vi "Set Worker.vi"(7 "Worker VI Path":path, 9 "State In":T1) -> (1 "State":T1, 2 "Is Worker?":bool)   [LabVIEW 2020, in "FlexBlock.xnode"]
uses:
  FlexBlock.xnode
  FlexBlocks/Terminal Direction.ctl
  FlexBlocks/FlexBlocks.lvlib
  FlexBlocks/Value Mode.ctl
  FlexBlocks/Terminal State.ctl
  FlexBlocks/Type Descriptor.ctl
  FlexBlocks/Errors.ctl
  <vilib>/picture/picture.llb/imagedata.ctl
  State.ctl
  FlexBlocks/Special Terminal.ctl
  FlexBlocks/Calculated Sizes.ctl
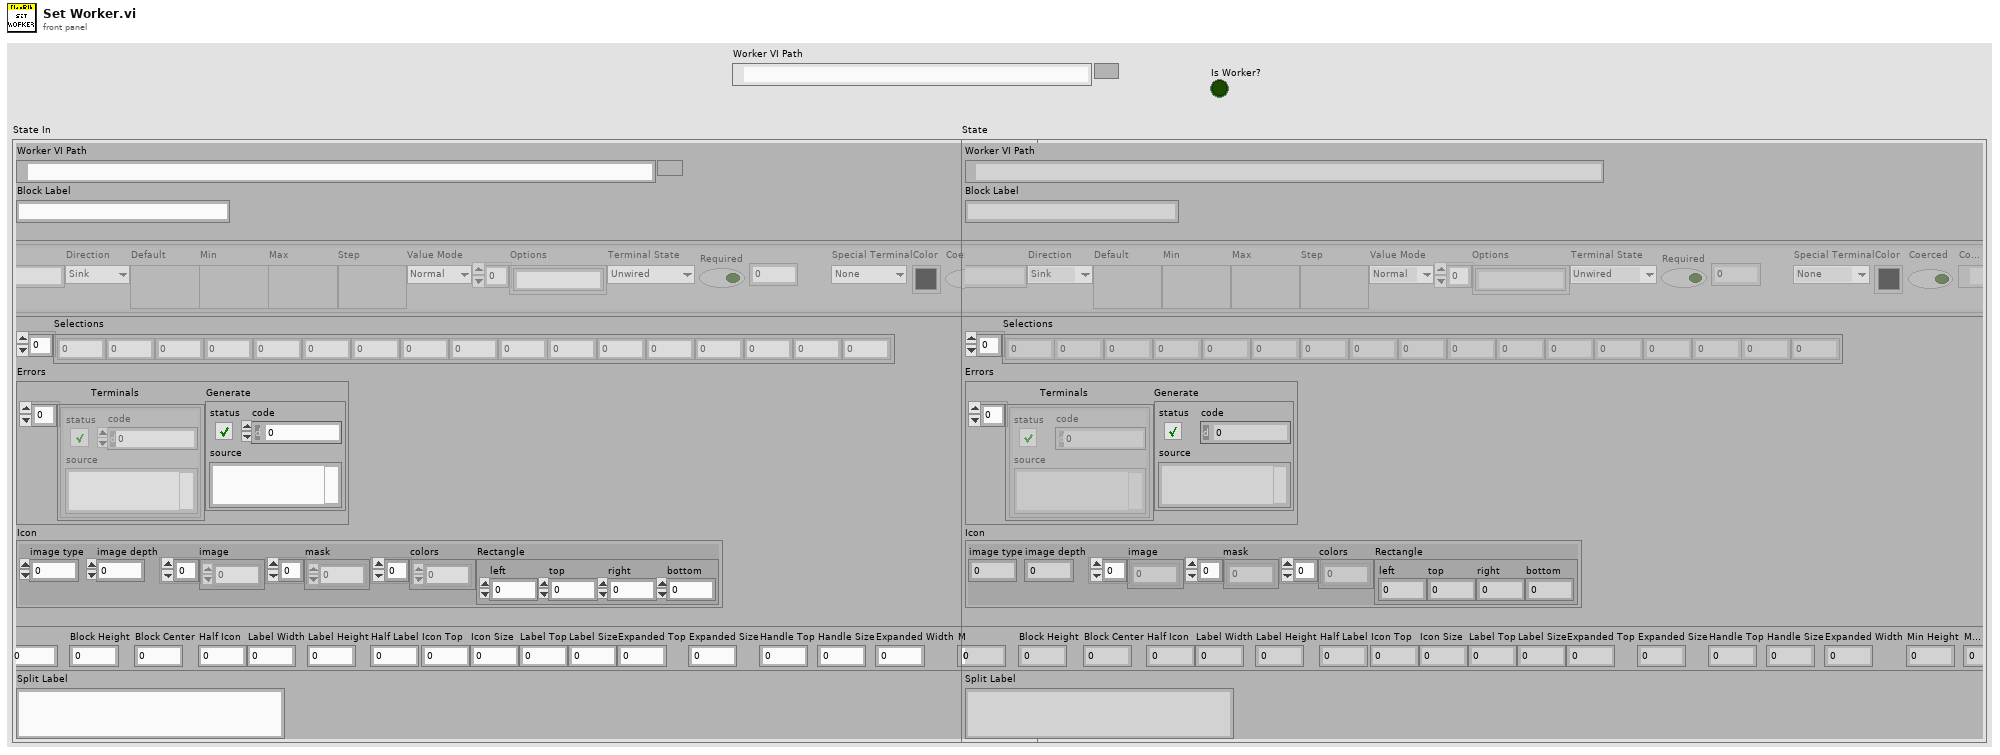
[diagram p1: front panel]
types:
  T1 = typedef "FlexBlock.xnode/State.ctl" = cluster{"Worker VI Path":path, "Block Label":string, "Types":T2[], "Selections":i32[], "Errors":T7, "Icon":T8, "Calcd Sizes":T9, "Split Label":string}
  T2 = typedef "FlexBlocks.lvlib/Type Descriptor.ctl" = cluster{"Name":string, "Direction":T3, "Default":variant, "Min":variant, "Max":variant, "Step":variant, "Value Mode":T4, "Options":string[], "Terminal State":T5, "Required":bool, "Connpane Index":i32, "Special Terminal":T6, "Color":u32, "Coerced":bool, "Connection Path":path}
  T3 = typedef "FlexBlocks.lvlib/Terminal Direction.ctl" = enum16{"Sink", "Source"}
  T4 = typedef "FlexBlocks.lvlib/Value Mode.ctl" = enum16{"Normal", "Range", "Select"}
  T5 = typedef "FlexBlocks.lvlib/Terminal State.ctl" = enum16{"Unwired", "BadType", "BadRef", "Channel", "Value", "Control Ref"}
  T6 = typedef "FlexBlocks.lvlib/Special Terminal.ctl" = enum16{"None", "Action", "Init", "Tag", "State in", "State out", "Error"}
  T7 = typedef "FlexBlocks.lvlib/Errors.ctl" = cluster{"Terminals":errorcluster[], "Generate":errorcluster}
  T8 = typedef "imagedata.ctl" = cluster{"image type":i32, "image depth":i32, "image":u8[], "mask":u8[], "colors":u32[], "Rectangle":cluster{"left":i16, "top":i16, "right":i16, "bottom":i16}}
  T9 = typedef "FlexBlocks.lvlib/Calculated Sizes.ctl" = cluster{"Text Width":i32, "Text Height":i32, "Half Text":i32, "Block Width":i32, "Block Height":i32, "Block Center":i32, "Half Icon":i32, "Label Width":i32, "Label Height":i32, "Half Label":i32, "Icon Top":i32, "Icon Size":i32, "Label Top":i32, "Label Size":i32, "Expanded Top":i32, "Expanded Size":i32, "Handle Top":i32, "Handle Size":i32, "Expanded Width":i32, "Min Height":i32, "Max Height":i32}
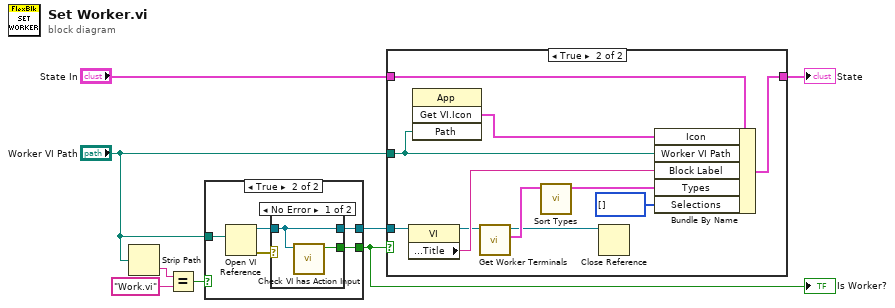
[diagram p0: block diagram]
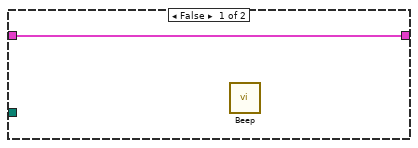
[diagram p2: hidden frame]
diagram:
  n1 = Strip Path(path="Worker VI Path") -> (name=w8:string)  [unwired: 1 out]
  n2 = Equal?(x=w8, y="Work.vi") -> (x = y?=w6:bool)
  n3 = case shown="True" w6 {
    tunnel: "Worker VI Path" -> [_ w13]
    tunnel: [_ w10] -> w4
    tunnel: [_ w9] -> w5
    frame False {
    }
    frame True {
      n4 = Open VI Reference(vi path=w13) -> (vi reference=w12:refnum<vi>, error out=w11:errorcluster)  [unwired: 5 in]
      n5 = case shown="No Error" w11 {
        tunnel: w12 -> [w14 _]
        tunnel: [w15 _] -> w10
        tunnel: [w14 _] -> w9
        frame No Error {
          n6 = call "Check VI has Action Input.vi"("Worker VI"=w14) -> ("Action Input?"=w15:bool)  [unwired: 10 in]
        }
        frame Error {
        }
      }
    }
  }
  "Is Worker?" <- w4
  n7 = case shown="True" w4 {
    tunnel: w5 -> [_ w27]
    tunnel: "State In" -> [w16 w26]
    tunnel: "Worker VI Path" -> [_ w24]
    tunnel: [w16 w18] -> w1
    frame False {
      n8 = call <vilib>:"Beep.vi"() -> ()  [unwired: 12 in]
    }
    frame True {
      n9 = property class="VI"(reference=w27) -> (reference out=w22:refnum<vi>, "Front Panel.Title"=w23:string)  [unwired: 1 in, 1 out]
      n10 = invoke class="App" method="Get VI.Icon"("Path"=w24) -> ("Get VI.Icon"=w25:T8)  [unwired: 3 in, 3 out]
      n11 = call "Get Worker Terminals.vi"("Worker VI"=w22) -> ("Types"=w21:T2[], "Worker VI out"=w19:refnum<vi>)  [unwired: 8 in, 1 out]
      n12 = call "Sort Types.vi"("Types"=w21) -> ("Sorted Types"=w17:T2[])  [unwired: 10 in]
      n13 = Close Reference(reference=w19) -> ()  [unwired: 1 in, 1 out]
      n14 = Bundle By Name(cluster=w26, "Icon"=w25, "Worker VI Path"=w24, "Block Label"=w23, "Types"=w17, "Selections"=i32[] []) -> (w18:T1)
    }
  }
  "State" <- w1
